vi "Measure.vi"(8 "error in (no error)":errorcluster, 11 "Hardware in":refnum<class "Hardware.lvclass">) -> (0 "error out":errorcluster, 2 "Measurement":dbl, 3 "Hardware out":refnum<class "Hardware.lvclass">)   [LabVIEW 2021, in "Hardware.lvclass"]
uses:
  Hardware.lvclass
  Hardware.lvclass/Hardware.ctl
  <vilib>/ptbypt/NI_PtbyPt.lvlib
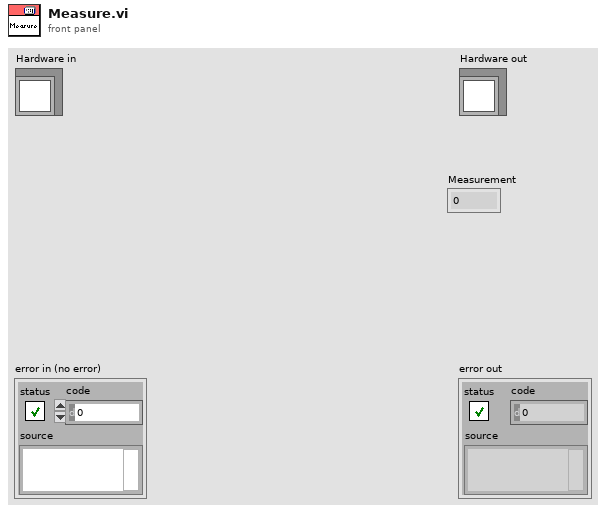
[diagram p1: front panel]
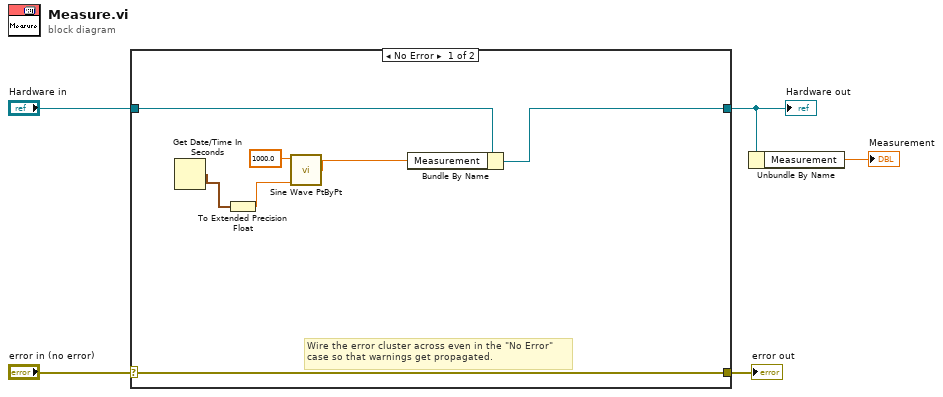
[diagram p0: block diagram]
diagram:
  n1 = case shown="No Error" "error in (no error)" {
    selector: "error in (no error)" -> [w12 w14]
    tunnel: [w12 w14] -> w4
    tunnel: [w11 w13] -> w2
    tunnel: "Hardware in" -> [w10 w13]
    frame No Error {
      # "Wire the error cluster across even in the \"No Error\"\ncase so that warnings get propagated."
      n2 = Get Date/Time In Seconds() -> (seconds since 1Jan1904=w7:timestamp)
      n3 = To Extended Precision Float(1:w7) -> (0:w6:ext)
      n4 = call <vilib>:"Sine Wave PtByPt.vi"("time"=w6, "amplitude"=1000.0) -> ("sine wave"=w9:dbl)  [unwired: 2 in]
      n5 = Bundle By Name(cluster=w10, "Measurement"=w9) -> (w11:refnum<class "Hardware.lvclass">)
    }
    frame Error {
    }
  }
  "error out" <- w4
  "Hardware out" <- w2
  n6 = Unbundle By Name(w2) -> ("Measurement"=→"Measurement":dbl)
